vi "Cycle 4 Main Spin Pause.vi"(0 "GEA2 Reference In":refnum<k24>, 1 "Basket Speeds (rpm)":u32[](array[numeric])=[125, 450, 700], 5 "GEA Inputs":T1={"Source"=228, "Destination"=35} {"Destination" format="%.0x"; "Source" format="%.0x"}, 7 "Standalone?":bool, 9 "Dwell Times (s)":dbl[](array[numeric])=[90.0, 30.0, 600.0], 11 "Error In":errorcluster, 12 "Basket Speed Tolerance (rpm)":u32=2) -> (4 "GEA2 Reference Out":refnum<k24>, 6 "Pass/Fail?":bool, 8 "Report Text":string, 15 "Error Out":errorcluster)   [LabVIEW 2016, in "TL27.lvlib"]
uses:
  Projects/TL27.lvlib
  C:/Automation/DLLs/PC Dot Net/GeaCommunication.dll
  Common/LabVIEW GEA2 Toolkit/LabVIEW_GEA2_Toolkit.lvlibp/type defs/Source_Destination.ctl
  Valew Common/type defs/Drive Cycle Engine Request State.ctl
  Common/LabVIEW GEA2 Toolkit/LabVIEW_GEA2_Toolkit.lvlibp/type defs/ERD Read Data In.ctl
  Common/LabVIEW GEA2 Toolkit/LabVIEW_GEA2_Toolkit.lvlibp/type defs/Data Type.ctl
  Common/LabVIEW GEA2 Toolkit/LabVIEW_GEA2_Toolkit.lvlibp
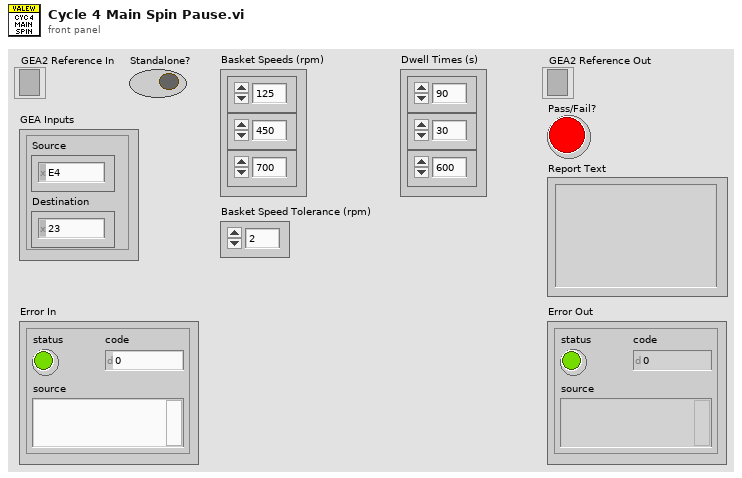
[diagram p1: front panel]
types:
  T1 = typedef "LabVIEW_GEA2_Toolkit.lvlibp/Source_Destination.ctl" = cluster{"Source":u8, "Destination":u8}
  T2 = typedef "TL27.lvlib/Drive Cycle Engine Request State.ctl" = enum16{"Start", "Stop", "Pause", "Resume", "Select"}
  T3 = typedef "LabVIEW_GEA2_Toolkit.lvlibp/ERD Read Data In.ctl" = cluster{"ERD Number":u16, "Data Type":T4}
  T4 = typedef "LabVIEW_GEA2_Toolkit.lvlibp/Data Type.ctl" = enum16{"string", "boolean", "uint8_t", "uint16_t", "uint32_t", "uint64_t", "int8_t", "int16_t", "int32_t", "int64_t"}
  T5 = typedef "LabVIEW_GEA2_Toolkit.lvlibp/ERD Read Data Out.ctl" = cluster{"ERD Number":u16, "Data":string}
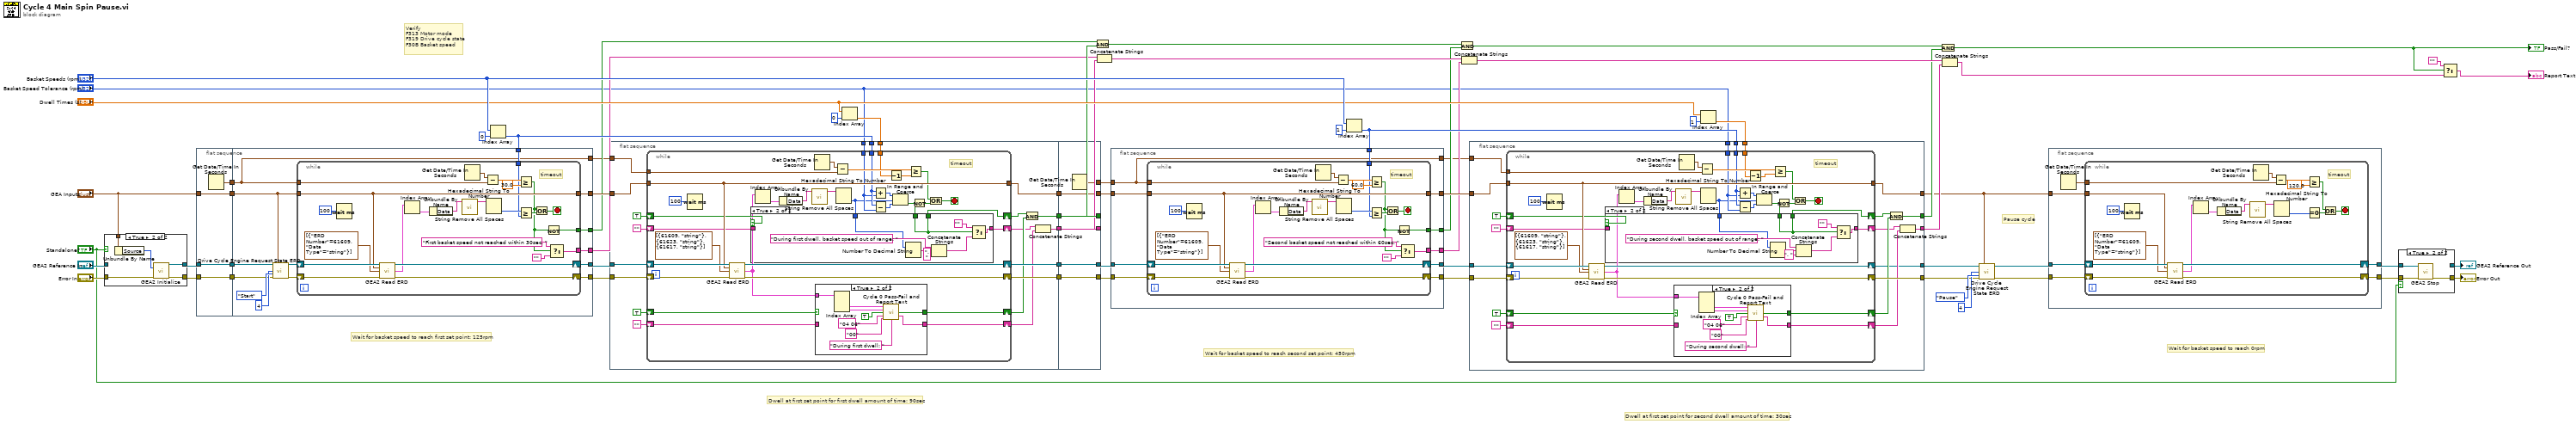
[diagram p0: block diagram]
diagram:
  # "Wait for basket speed to reach 0rpm"
  # "Pause cycle"
  # "Dwell at first set point for second dwell amount of time: 30sec"
  # "Wait for basket speed to reach second set point: 450rpm"
  # "Verify\nF313 Motor mode\nF319 Drive cycle state\nF30B Basket speed"
  # "Dwell at first set point for first dwell amount of time: 90sec"
  # "Wait for basket speed to reach first set point: 125rpm"
  n1 = case shown="True" "Standalone?" {
    tunnel: "GEA2 Reference In" -> [w67 _]
    tunnel: [w67 w72] -> w21
    tunnel: "Error In" -> [w66 w71]
    tunnel: [w66 w70] -> w22
    tunnel: "GEA Inputs" -> [_ w69]
    frame False {
    }
    frame True {
      n2 = Unbundle By Name(w69) -> ("Source"=w68:u8)
      n3 = call "GEA2 Initialize.vi"("Source Address"=w68, "error in"=w71) -> ("GEA2 Reference Out"=w72:refnum<k24>, "error out"=w70:errorcluster)  [unwired: 11 in, 1 out]
    }
  }
  n4 = flat-sequence {
    tunnel: "GEA Inputs" -> [w76]
    tunnel: [w76] -> w23
    tunnel: w22 -> [w73]
    tunnel: w21 -> [w74]
    tunnel: [w75] -> w20
    tunnel: [w74] -> w19
    tunnel: [w73] -> w18
    tunnel: [w90] -> w55
    tunnel: [w89] -> w56
    tunnel: [w88] -> w65
    tunnel: [w85] -> w37
    tunnel: [w86] -> w35
    tunnel: w44 -> [w87]
    tunnel: [w77] -> w25
    tunnel: w23 -> [w78]
    tunnel: w20 -> [w77]
    tunnel: w19 -> [w82]
    tunnel: w18 -> [w81]
    frame #0 {
      n5 = Get Date/Time In Seconds() -> (seconds since 1Jan1904=w75:timestamp)
    }
    frame #1 {
      n6 = call "Drive Cycle Engine Request State ERD.vi"("GEA2 Reference In"=w82, "GEA Inputs"=w78, "Cycle ID"=u8 4, "Drive Cycle Engine Request State"=Drive_Cycle_Engine_Request_State."Start", "Error In"=w81) -> ("GEA2 Reference Out"=w80:refnum<k24>, "Error Out"=w79:errorcluster)  [unwired: 9 in]
      n7 = while {
        shift-right: [w113] -> w90
        shift-left: w79 -> [w114]
        shift-right: [w111] -> w89
        shift-left: w80 -> [w112]
        tunnel: w78 -> [w109]
        tunnel: [w109] -> w88
        tunnel: w77 -> [w91]
        tunnel: w87 -> [w99]
        tunnel: [w94] -> w86
        tunnel: [w92] -> w85
        stop <- w106 stop-if-true
        # "timeout"
        n8 = Wait (ms)(milliseconds to wait=u32 100) -> ()  [unwired: 1 out]
        n9 = call "GEA2 Read ERD.vi"("GEA2 Reference In"=w112, "GEA Inputs"=w109, "Read ERD List"=T3[] [{"ERD Number"=61609, "Data Type"=enum."string"}], "Error In"=w114) -> ("GEA2 Reference Out"=w111:refnum<k24>, "ERD Data Out"=w98:T5[], "Error Out"=w113:errorcluster)  [unwired: 8 in, 1 out]
        n10 = Index Array(array=w98) -> (element=w110:T5)  [unwired: 1 in]
        n11 = Unbundle By Name(w110) -> ("Data"=w102:string)
        n12 = call "String Remove All Spaces.vi"("Input String"=w102) -> ("Spaces Removed"=w103:string)  [unwired: 13 in, 1 out]
        n13 = Get Date/Time In Seconds() -> (seconds since 1Jan1904=w107:timestamp)
        n14 = Subtract(x=w107, y=w91) -> (x-y=w108:dbl)
        n15 = Hexadecimal String To Number(string=w103) -> (number=w101:u32)  [unwired: 2 in, 1 out]
        n16 = Greater Or Equal?(x=w108, y=30.0) -> (x >= y?=w93:bool)
        n17 = Greater Or Equal?(x=w101, y=w99) -> (x >= y?=w97:bool)
        n18 = Or(x=w93, y=w97) -> (x .or. y?=w106:bool)
        n19 = Not(x=w93) -> (.not. x?=w92:bool)
        n20 = Select(t="First basket speed not reached within 30sec. ", s=w93, f="") -> (s? t:f=w94:string)
      }
    }
  }
  n21 = Index Array(array="Basket Speeds (rpm)", index=0) -> (element=w44:u32)
  n22 = flat-sequence {
    tunnel: w58 -> [w127]
    tunnel: w44 -> [w126]
    tunnel: "Basket Speed Tolerance (rpm)" -> [w125]
    tunnel: w55 -> [w132]
    tunnel: w65 -> [w133]
    tunnel: w56 -> [w134]
    tunnel: w25 -> [w115]
    tunnel: [w130] -> w14
    tunnel: [w129] -> w13
    tunnel: [w128] -> w12
    tunnel: [w119] -> w11
    tunnel: [w116] -> w10
    tunnel: [w189] -> w15
    tunnel: [w190] -> w34
    tunnel: [w191] -> w36
    tunnel: [w192] -> w52
    tunnel: [w193] -> w54
    tunnel: [w194] -> w53
    tunnel: w14 -> [w194]
    tunnel: w13 -> [w193]
    tunnel: w12 -> [w192]
    tunnel: w11 -> [w191]
    tunnel: w10 -> [w190]
    frame #0 {
      n23 = while {
        shift-right: [w166] -> w130
        shift-left: w132 -> [w167]
        shift-right: [w164] -> w129
        shift-left: w134 -> [w165]
        tunnel: w133 -> [w162]
        tunnel: [w162] -> w128
        tunnel: w115 -> [w160]
        shift-right: [w144] -> w120
        shift-left: TRUE -> [w146]
        tunnel: w127 -> [w136]
        tunnel: w126 -> [w151]
        tunnel: w125 -> [w150]
        shift-right: [w148] -> w117
        shift-left: "" -> [w145]
        shift-right: [w138] -> w121
        shift-left: TRUE -> [w141]
        shift-right: [w139] -> w118
        shift-left: "" -> [w140]
        stop <- w158 stop-if-true
        # "timeout"
        n24 = Wait (ms)(milliseconds to wait=u32 100) -> ()  [unwired: 1 out]
        n25 = call "GEA2 Read ERD.vi"("GEA2 Reference In"=w165, "GEA Inputs"=w162, "Read ERD List"=T3[] [{"ERD Number"=61609, "Data Type"=enum."string"}, {"ERD Number"=61623, "Data Type"=enum."string"}, {"ERD Number"=61617, "Data Type"=enum."string"}], "Error In"=w167) -> ("GEA2 Reference Out"=w164:refnum<k24>, "ERD Data Out"=w137:T5[], "Error Out"=w166:errorcluster)  [unwired: 8 in, 1 out]
        n26 = Index Array(array=w137) -> (element=w163:T5)  [unwired: 1 in]
        n27 = Unbundle By Name(w163) -> ("Data"=w154:string)
        n28 = call "String Remove All Spaces.vi"("Input String"=w154) -> ("Spaces Removed"=w155:string)  [unwired: 13 in, 1 out]
        n29 = Get Date/Time In Seconds() -> (seconds since 1Jan1904=w159:timestamp)
        n30 = case shown="True" w141 {
          selector: w141 -> [w168 _]
          tunnel: w140 -> [w169 _]
          tunnel: [w169 w177] -> w139
          tunnel: [w168 w178] -> w138
          tunnel: w137 -> [_ w176]
          frame False {
          }
          frame True {
            n31 = Index Array(array=w176) -> (element #2=w174:T5, element #3=w173:T5)  [unwired: 3 in, 1 out]
            n32 = call "Cycle 0 Pass-Fail and Report Text.vi"("Drive Cycle State"=w174, "Motor Mode"=w173, "Previous Pass/Fail"=TRUE, "Cycle State Expected"="04 06", "Motor Mode Expected"="00", "Header"="During first dwell: ") -> ("Pass/Fail?"=w178:bool, "Report Text"=w177:string)  [unwired: 8 in]
          }
        }
        n33 = Subtract(x=w159, y=w160) -> (x-y=w161:dbl)
        n34 = Hexadecimal String To Number(string=w155) -> (number=w149:u32)  [unwired: 2 in, 1 out]
        n35 = Add(x=w151, y=w150) -> (x+y=w153:u32)
        n36 = Subtract(x=w151, y=w150) -> (x-y=w152:u32)
        n37 = Decrement(x=w136) -> (x-1=w135:dbl)
        n38 = In Range and Coerce(upper limit=w153, x=w149, lower limit=w152) -> (In Range?=w147:bool)  [unwired: 1 out]
        n39 = case shown="True" w146 {
          selector: w146 -> [w179 _]
          tunnel: w149 -> [_ w186]
          tunnel: [w180 w183] -> w148
          tunnel: w147 -> [_ w182]
          tunnel: w145 -> [w180 _]
          tunnel: [w179 w182] -> w144
          frame False {
          }
          frame True {
            n40 = Number To Decimal String(number=w186) -> (decimal integer string=w185:string)  [unwired: 1 in]
            n41 = Concatenate Strings("During first dwell, basket speed out of range: " ("string"), w185, ". " ("string")) -> (w184:string)
            n42 = Select(t="", s=w182, f=w184) -> (s? t:f=w183:string)
          }
        }
        n43 = Greater Or Equal?(x=w161, y=w135) -> (x >= y?=w142:bool)
        n44 = Not(x=w147) -> (.not. x?=w143:bool)
        n45 = Or(x=w142, y=w143) -> (x .or. y?=w158:bool)
      }
      n46 = And(x=w120, y=w121) -> (x .and. y?=w119:bool)
      n47 = Concatenate Strings(w117, w118) -> (w116:string)
    }
    frame #1 {
      n48 = Get Date/Time In Seconds() -> (seconds since 1Jan1904=w189:timestamp)
    }
  }
  n49 = Index Array(array="Dwell Times (s)", index=0) -> (element=w58:dbl)
  n50 = And(x=w37, y=w36) -> (x .and. y?=w33:bool)
  n51 = Concatenate Strings(w35, w34) -> (w32:string)
  n52 = flat-sequence {
    tunnel: [w201] -> w50
    tunnel: [w200] -> w49
    tunnel: [w199] -> w48
    tunnel: [w196] -> w30
    tunnel: [w197] -> w31
    tunnel: w47 -> [w198]
    tunnel: w53 -> [w202]
    tunnel: w52 -> [w203]
    tunnel: w54 -> [w204]
    tunnel: [w195] -> w24
    tunnel: w15 -> [w195]
    frame #0 {
      n53 = while {
        shift-right: [w227] -> w201
        shift-left: w202 -> [w228]
        shift-right: [w225] -> w200
        shift-left: w204 -> [w226]
        tunnel: w203 -> [w223]
        tunnel: [w223] -> w199
        tunnel: w195 -> [w205]
        tunnel: w198 -> [w213]
        tunnel: [w208] -> w197
        tunnel: [w206] -> w196
        stop <- w220 stop-if-true
        # "timeout"
        n54 = Wait (ms)(milliseconds to wait=u32 100) -> ()  [unwired: 1 out]
        n55 = call "GEA2 Read ERD.vi"("GEA2 Reference In"=w226, "GEA Inputs"=w223, "Read ERD List"=T3[] [{"ERD Number"=61609, "Data Type"=enum."string"}], "Error In"=w228) -> ("GEA2 Reference Out"=w225:refnum<k24>, "ERD Data Out"=w212:T5[], "Error Out"=w227:errorcluster)  [unwired: 8 in, 1 out]
        n56 = Index Array(array=w212) -> (element=w224:T5)  [unwired: 1 in]
        n57 = Unbundle By Name(w224) -> ("Data"=w216:string)
        n58 = call "String Remove All Spaces.vi"("Input String"=w216) -> ("Spaces Removed"=w217:string)  [unwired: 13 in, 1 out]
        n59 = Get Date/Time In Seconds() -> (seconds since 1Jan1904=w221:timestamp)
        n60 = Subtract(x=w221, y=w205) -> (x-y=w222:dbl)
        n61 = Hexadecimal String To Number(string=w217) -> (number=w215:u32)  [unwired: 2 in, 1 out]
        n62 = Greater Or Equal?(x=w222, y=60.0) -> (x >= y?=w207:bool)
        n63 = Greater Or Equal?(x=w215, y=w213) -> (x >= y?=w211:bool)
        n64 = Or(x=w207, y=w211) -> (x .or. y?=w220:bool)
        n65 = Not(x=w207) -> (.not. x?=w206:bool)
        n66 = Select(t="Second basket speed not reached within 60sec. ", s=w207, f="") -> (s? t:f=w208:string)
      }
    }
  }
  n67 = Index Array(array="Basket Speeds (rpm)", index=1) -> (element=w47:u32)
  n68 = And(x=w33, y=w30) -> (x .and. y?=w27:bool)
  n69 = Concatenate Strings(w32, w31) -> (w28:string)
  n70 = flat-sequence {
    tunnel: [w244] -> w38
    tunnel: [w243] -> w1
    tunnel: [w234] -> w26
    tunnel: [w231] -> w29
    tunnel: w45 -> [w242]
    tunnel: w47 -> [w241]
    tunnel: "Basket Speed Tolerance (rpm)" -> [w240]
    tunnel: w50 -> [w246]
    tunnel: w48 -> [w247]
    tunnel: w49 -> [w248]
    tunnel: [w230] -> w39
    tunnel: w24 -> [w229]
    frame #0 {
      n71 = while {
        shift-right: [w280] -> w244
        shift-left: w246 -> [w281]
        shift-right: [w278] -> w230
        shift-left: w248 -> [w279]
        tunnel: w247 -> [w276]
        tunnel: [w276] -> w243
        tunnel: w229 -> [w274]
        shift-right: [w258] -> w235
        shift-left: TRUE -> [w260]
        tunnel: w242 -> [w250]
        tunnel: w241 -> [w265]
        tunnel: w240 -> [w264]
        shift-right: [w262] -> w232
        shift-left: "" -> [w259]
        shift-right: [w252] -> w236
        shift-left: TRUE -> [w255]
        shift-right: [w253] -> w233
        shift-left: "" -> [w254]
        stop <- w272 stop-if-true
        # "timeout"
        n72 = Wait (ms)(milliseconds to wait=u32 100) -> ()  [unwired: 1 out]
        n73 = call "GEA2 Read ERD.vi"("GEA2 Reference In"=w279, "GEA Inputs"=w276, "Read ERD List"=T3[] [{"ERD Number"=61609, "Data Type"=enum."string"}, {"ERD Number"=61623, "Data Type"=enum."string"}, {"ERD Number"=61617, "Data Type"=enum."string"}], "Error In"=w281) -> ("GEA2 Reference Out"=w278:refnum<k24>, "ERD Data Out"=w251:T5[], "Error Out"=w280:errorcluster)  [unwired: 8 in, 1 out]
        n74 = Index Array(array=w251) -> (element=w277:T5)  [unwired: 1 in]
        n75 = Unbundle By Name(w277) -> ("Data"=w268:string)
        n76 = case shown="True" w255 {
          selector: w255 -> [w282 _]
          tunnel: w254 -> [w283 _]
          tunnel: [w283 w291] -> w253
          tunnel: [w282 w292] -> w252
          tunnel: w251 -> [_ w290]
          frame False {
          }
          frame True {
            n77 = Index Array(array=w290) -> (element #2=w288:T5, element #3=w287:T5)  [unwired: 3 in, 1 out]
            n78 = call "Cycle 0 Pass-Fail and Report Text.vi"("Drive Cycle State"=w288, "Motor Mode"=w287, "Previous Pass/Fail"=TRUE, "Cycle State Expected"="04 06", "Motor Mode Expected"="00", "Header"="During second dwell: ") -> ("Pass/Fail?"=w292:bool, "Report Text"=w291:string)  [unwired: 8 in]
          }
        }
        n79 = call "String Remove All Spaces.vi"("Input String"=w268) -> ("Spaces Removed"=w269:string)  [unwired: 13 in, 1 out]
        n80 = Get Date/Time In Seconds() -> (seconds since 1Jan1904=w273:timestamp)
        n81 = Subtract(x=w273, y=w274) -> (x-y=w275:dbl)
        n82 = Hexadecimal String To Number(string=w269) -> (number=w263:u32)  [unwired: 2 in, 1 out]
        n83 = Add(x=w265, y=w264) -> (x+y=w267:u32)
        n84 = Subtract(x=w265, y=w264) -> (x-y=w266:u32)
        n85 = Decrement(x=w250) -> (x-1=w249:dbl)
        n86 = In Range and Coerce(upper limit=w267, x=w263, lower limit=w266) -> (In Range?=w261:bool)  [unwired: 1 out]
        n87 = case shown="True" w260 {
          selector: w260 -> [w293 _]
          tunnel: w263 -> [_ w300]
          tunnel: [w294 w297] -> w262
          tunnel: w261 -> [_ w296]
          tunnel: w259 -> [w294 _]
          tunnel: [w293 w296] -> w258
          frame False {
          }
          frame True {
            n88 = Number To Decimal String(number=w300) -> (decimal integer string=w299:string)  [unwired: 1 in]
            n89 = Concatenate Strings("During second dwell, basket speed out of range: " ("string"), w299, ". " ("string")) -> (w298:string)
            n90 = Select(t="", s=w296, f=w298) -> (s? t:f=w297:string)
          }
        }
        n91 = Greater Or Equal?(x=w275, y=w249) -> (x >= y?=w256:bool)
        n92 = Not(x=w261) -> (.not. x?=w257:bool)
        n93 = Or(x=w256, y=w257) -> (x .or. y?=w272:bool)
      }
      n94 = And(x=w235, y=w236) -> (x .and. y?=w234:bool)
      n95 = Concatenate Strings(w232, w233) -> (w231:string)
    }
  }
  n96 = Index Array(array="Dwell Times (s)", index=1) -> (element=w45:dbl)
  n97 = And(x=w27, y=w26) -> (x .and. y?=w6:bool)
  "Pass/Fail?" <- w6
  n98 = Concatenate Strings(w28, w29) -> (w7:string)
  n99 = call "Drive Cycle Engine Request State ERD.vi"("GEA2 Reference In"=w39, "GEA Inputs"=w1, "Cycle ID"=u8 4, "Drive Cycle Engine Request State"=Drive_Cycle_Engine_Request_State."Pause", "Error In"=w38) -> ("GEA2 Reference Out"=w9:refnum<k24>, "Error Out"=w8:errorcluster)  [unwired: 9 in]
  n100 = flat-sequence {
    tunnel: [w307] -> w4
    tunnel: [w306] -> w5
    tunnel: w9 -> [w305]
    tunnel: w8 -> [w304]
    tunnel: w1 -> [w303]
    frame #0 {
      n101 = Get Date/Time In Seconds() -> (seconds since 1Jan1904=w308:timestamp)
      n102 = while {
        shift-right: [w326] -> w307
        shift-left: w304 -> [w327]
        shift-right: [w324] -> w306
        shift-left: w305 -> [w325]
        tunnel: w308 -> [w310]
        tunnel: w303 -> [w309]
        stop <- w320 stop-if-true
        # "timeout"
        n103 = Wait (ms)(milliseconds to wait=u32 100) -> ()  [unwired: 1 out]
        n104 = call "GEA2 Read ERD.vi"("GEA2 Reference In"=w325, "GEA Inputs"=w309, "Read ERD List"=T3[] [{"ERD Number"=61609, "Data Type"=enum."string"}], "Error In"=w327) -> ("GEA2 Reference Out"=w324:refnum<k24>, "ERD Data Out"=w313:T5[], "Error Out"=w326:errorcluster)  [unwired: 8 in, 1 out]
        n105 = Index Array(array=w313) -> (element=w323:T5)  [unwired: 1 in]
        n106 = Unbundle By Name(w323) -> ("Data"=w316:string)
        n107 = call "String Remove All Spaces.vi"("Input String"=w316) -> ("Spaces Removed"=w317:string)  [unwired: 13 in, 1 out]
        n108 = Get Date/Time In Seconds() -> (seconds since 1Jan1904=w321:timestamp)
        n109 = Subtract(x=w321, y=w310) -> (x-y=w322:dbl)
        n110 = Hexadecimal String To Number(string=w317) -> (number=w315:u32)  [unwired: 2 in, 1 out]
        n111 = Greater Or Equal?(x=w322, y=120.0) -> (x >= y?=w311:bool)
        n112 = Equal To 0?(x=w315) -> (x = 0?=w312:bool)
        n113 = Or(x=w311, y=w312) -> (x .or. y?=w320:bool)
      }
    }
  }
  n114 = case shown="True" "Standalone?" {
    tunnel: [w328 w332] -> w62
    tunnel: w4 -> [w328 w331]
    tunnel: w5 -> [w329 w330]
    tunnel: [w329 _] -> w61
    frame False {
    }
    frame True {
      n115 = call "GEA2 Stop.vi"("GEA2 Reference In"=w330, "Error In"=w331) -> ("Error Out"=w332:errorcluster)  [unwired: 13 in]
    }
  }
  "GEA2 Reference Out" <- w61
  "Error Out" <- w62
  n116 = Select(t="", s=w6, f=w7) -> (s? t:f=→"Report Text":string)
